vi "database input.vi"(4 "Wheel Name":string="cycle results testdbrunorder.txt", 6 "run number":string="46", 7 "wheelnumber":string, 8 "error in (no error)":errorcluster, 9 "readouts string":string="\r\n1/4/2012 10:09:06 AM\t103752\tWeavCaMB11\tb\tJackson\t0\t3\t50\t1231.000000\tInf\t35.314700\t5.667000\t336.000000\t0.988235\t3599.788248\t31.964787\t6135967.567040\t26573.858939\t1411896.374545\t0.000620\t59.996471\t23532.990455\tNaN\tInf\t0.000000\tNaN\t0.000000\t879579.012026\tNaN\t26573.858939\t0.433083\tNaN\tNaN\tNaN\t7.758172", 10 "runletter":string="testwheellllll", 11 "beamline readbacks":T6={"Injector"=[0.023339, 0.023338, 0.023336000000000003, 0.023338, 0.023336000000000003, 0.023336000000000003, 0.023334], "Analyze"=[0.0058, 0.0058, 0.0058, 0.0058, 0.0058, 0.0058, 0.0058], "Switch"=[0.0, 0.0, 0.0, 0.0, 0.0, 0.0, 0.0], "Terminal"=[0.0010328292846679688, 0.0010328292846679688, 0.0013613700866699219, 0.0007047653198242188, 0.0010328292846679688, 0.0010328292846679688, 0.0010328292846679688], "Cathode"=[10.239062309265137, 10.239218711853027, 10.239218711853027, 10.239218711853027, 10.239218711853027, 10.239218711853027, 10.239218711853027]}) -> (0 "error out":errorcluster={"status"=TRUE, "code"=-2147467259, "source"="NI_Database_API.lvlib:Cmd Execute.vi->NI_Database_API.lvlib:DB Tools Insert Data.vi->database input.vi->2d ams run o17.vi<ERR>ADO Error: 0x80004005\r\nException occured in Microsoft OLE DB Provider for ODBC Drivers: ERROR: invalid input syntax for type double precision: \"True\";\nError while executing the query in NI_Database_API.lvlib:Rec Create - Command.vi->NI_Database_API.lvlib:Cmd Execute.vi->NI_Database_API.lvlib:DB Tools Insert Data.vi->database input.vi->2d ams run o17.vi"}, 1 "db cluster":T5={"startat"="\r\n1/4/2012 10:09:06 AM", "holderid"="103752", "Sample Name"="WeavCaMB11", "type"="b", "User Name"="Jackson", "cycle measured"="0", "position"="3", "estimated ratio"="50", "cycle"="1231.000000", "Transmission"="Inf", "first currents"="35.314700", "runtime"="5.667000", "total rare counts"="336.000000", "livetime"="0.988235", "Rare CPM"="3599.788248", "second current"="31.964787", "17O ratio"="6135967.567040", "17O error"="26573.858939", "Cycle Ratio"="1411896.374545", "cycle error"="0.000620", "interference"="59.996471", "use"="True", "InjSS"="NaN", "He SS"="Inf", "Oaverage"="0.000000", "wheelnumber"="46", "wheel name"="cycle results testdbrunorder.txt", "runnumber"="{0.023339,0.023338,0.023336,0.023338,0.023336,0.023336,0.023334\r\n}", "runletter"="{0.005800,0.005800,0.005800,0.005800,0.005800,0.005800,0.005800\r\n}", "runletter 2"="{0.000000,0.000000,0.000000,0.000000,0.000000,0.000000,0.000000\r\n}"})   [LabVIEW 2016]
doc: "inputs data into cycleresults table in database"
uses:
  controls/db cluster.ctl
  <vilib>/addons/database/Connection.llb/DB Tools Open Connec (String).vi
  <vilib>/addons/database/NI_Database_API.lvlib
panel:
  out "cluster 2":T1
  out "cluster":T2
  out "output cluster 2":T3
  out "output cluster":T4
  in  "db cluster 2":T5={"startat"="\r\n1/4/2012 10:09:06 AM", "holderid"="103752", "Sample Name"="WeavCaMB11", "type"="b", "User Name"="Jackson", "cycle measured"="0", "position"="3", "estimated ratio"="50", "cycle"="1231.000000", "Transmission"="Inf", "first currents"="35.314700", "runtime"="5.667000", "total rare counts"="336.000000", "livetime"="0.988235", "Rare CPM"="3599.788248", "second current"="31.964787", "17O ratio"="6135967.567040", "17O error"="26573.858939", "Cycle Ratio"="1411896.374545", "cycle error"="0.000620", "interference"="59.996471", "use"="True", "InjSS"="NaN", "He SS"="Inf", "Oaverage"="0.000000", "wheelnumber"="46", "wheel name"="cycle results testdbrunorder.txt", "runnumber"="{0.023339,0.023338,0.023336,0.023338,0.023336,0.023336,0.023334\r\n}", "runletter"="{0.005800,0.005800,0.005800,0.005800,0.005800,0.005800,0.005800\r\n}", "runletter 2"="{0.000000,0.000000,0.000000,0.000000,0.000000,0.000000,0.000000\r\n}"}
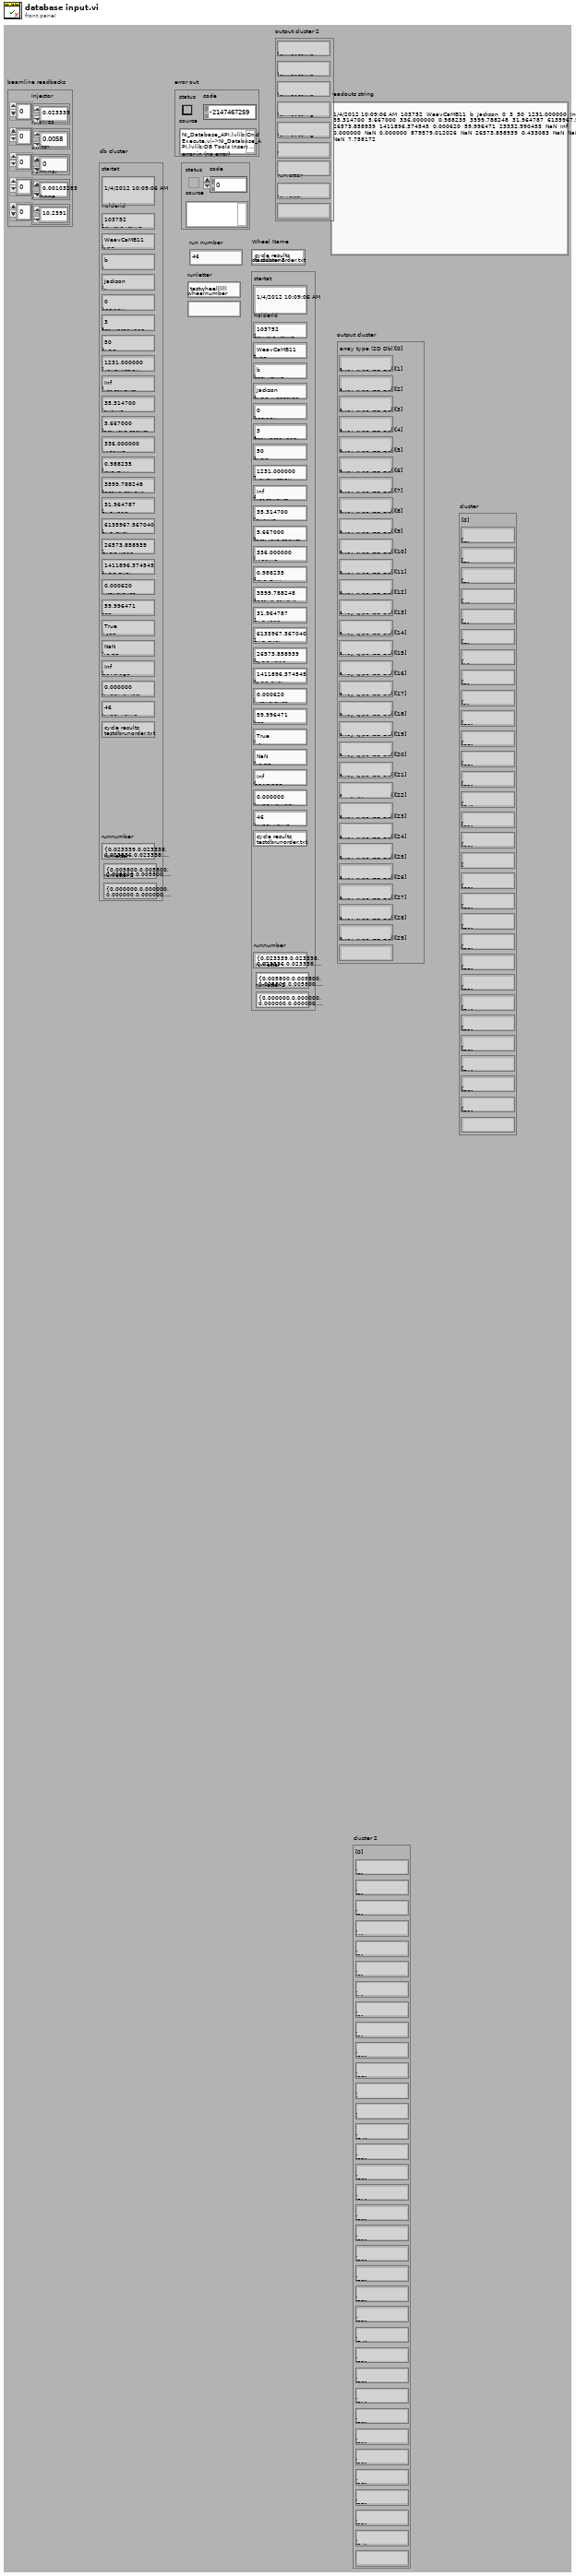
[diagram p1: front panel]
types:
  T1 = cluster{"[0]":string, "[1]":string, "[2]":string, "[3]":string, "[4]":string, "[5]":string, "[6]":string, "[7]":string, "[8]":string, "[9]":string, "[10]":string, "[11]":string, "[12]":string, "[13]":string, "[14]":string, "[15]":string, "[16]":string, "[17]":string, "[18]":string, "[19]":string, "[20]":string, "[21]":string, "[22]":string, "[23]":string, "[24]":string, "[25]":string, "[26]":string, "[27]":string, "[28]":string, "[29]":string, "[30]":string, "[31]":string, "[32]":string, "[33]":string, "[34]":string}
  T2 = cluster{"[0]":string, "[1]":string, "[2]":string, "[3]":string, "[4]":string, "[5]":string, "[6]":string, "[7]":string, "[8]":string, "[9]":string, "[10]":string, "[11]":string, "[12]":string, "[13]":string, "[14]":string, "[15]":string, "[16]":string, "[17]":string, "[18]":string, "[19]":string, "[20]":string, "[21]":string, "[22]":string, "[23]":string, "[24]":string, "[25]":string, "[26]":string, "[27]":string, "[28]":string, "[29]":string}
  T3 = cluster{string, "format string":string, "format string":string, "format string":string, "format string":string, "format string":string, "Wheel Number":string, "runletter":string, "runletter":string}
  T4 = cluster{"array type (2D Dbl)[0]":string, "array type (2D Dbl)[1]":string, "array type (2D Dbl)[2]":string, "array type (2D Dbl)[3]":string, "array type (2D Dbl)[4]":string, "array type (2D Dbl)[5]":string, "array type (2D Dbl)[6]":string, "array type (2D Dbl)[7]":string, "array type (2D Dbl)[8]":string, "array type (2D Dbl)[9]":string, "array type (2D Dbl)[10]":string, "array type (2D Dbl)[11]":string, "array type (2D Dbl)[12]":string, "array type (2D Dbl)[13]":string, "array type (2D Dbl)[14]":string, "array type (2D Dbl)[15]":string, "array type (2D Dbl)[16]":string, "array type (2D Dbl)[17]":string, "array type (2D Dbl)[18]":string, "array type (2D Dbl)[19]":string, "array type (2D Dbl)[20]":string, "array type (2D Dbl)[21]":string, "array type (2D Dbl)[22]":string, "array type (2D Dbl)[23]":string, "array type (2D Dbl)[24]":string, "array type (2D Dbl)[25]":string, "array type (2D Dbl)[26]":string, "array type (2D Dbl)[27]":string, "array type (2D Dbl)[28]":string, "array type (2D Dbl)[29]":string}
  T5 = typedef "db cluster.ctl" = cluster{"startat":string, "holderid":string, "Sample Name":string, "type":string, "User Name":string, "cycle measured":string, "position":string, "estimated ratio":string, "cycle":string, "Transmission":string, "first currents":string, "runtime":string, "total rare counts":string, "livetime":string, "Rare CPM":string, "second current":string, "17O ratio":string, "17O error":string, "Cycle Ratio":string, "cycle error":string, "interference":string, "use":string, "InjSS":string, "He SS":string, "Oaverage":string, "wheelnumber":string, "wheel name":string, "runnumber":string, "runletter":string, "runletter 2":string}
  T6 = cluster{"Injector":dbl[], "Analyze":dbl[], "Switch":dbl[], "Terminal":dbl[], "Cathode":dbl[]}
  T7 = cluster{string, "format string":string, "format string":string, "format string":string, "format string":string, "format string":string, "wheelnumber":string, "runletter":string, "run number":string}
  T8 = typedef "NI_Database_API.lvlib/Conn ObjectReference.ctl" = refnum<k1>
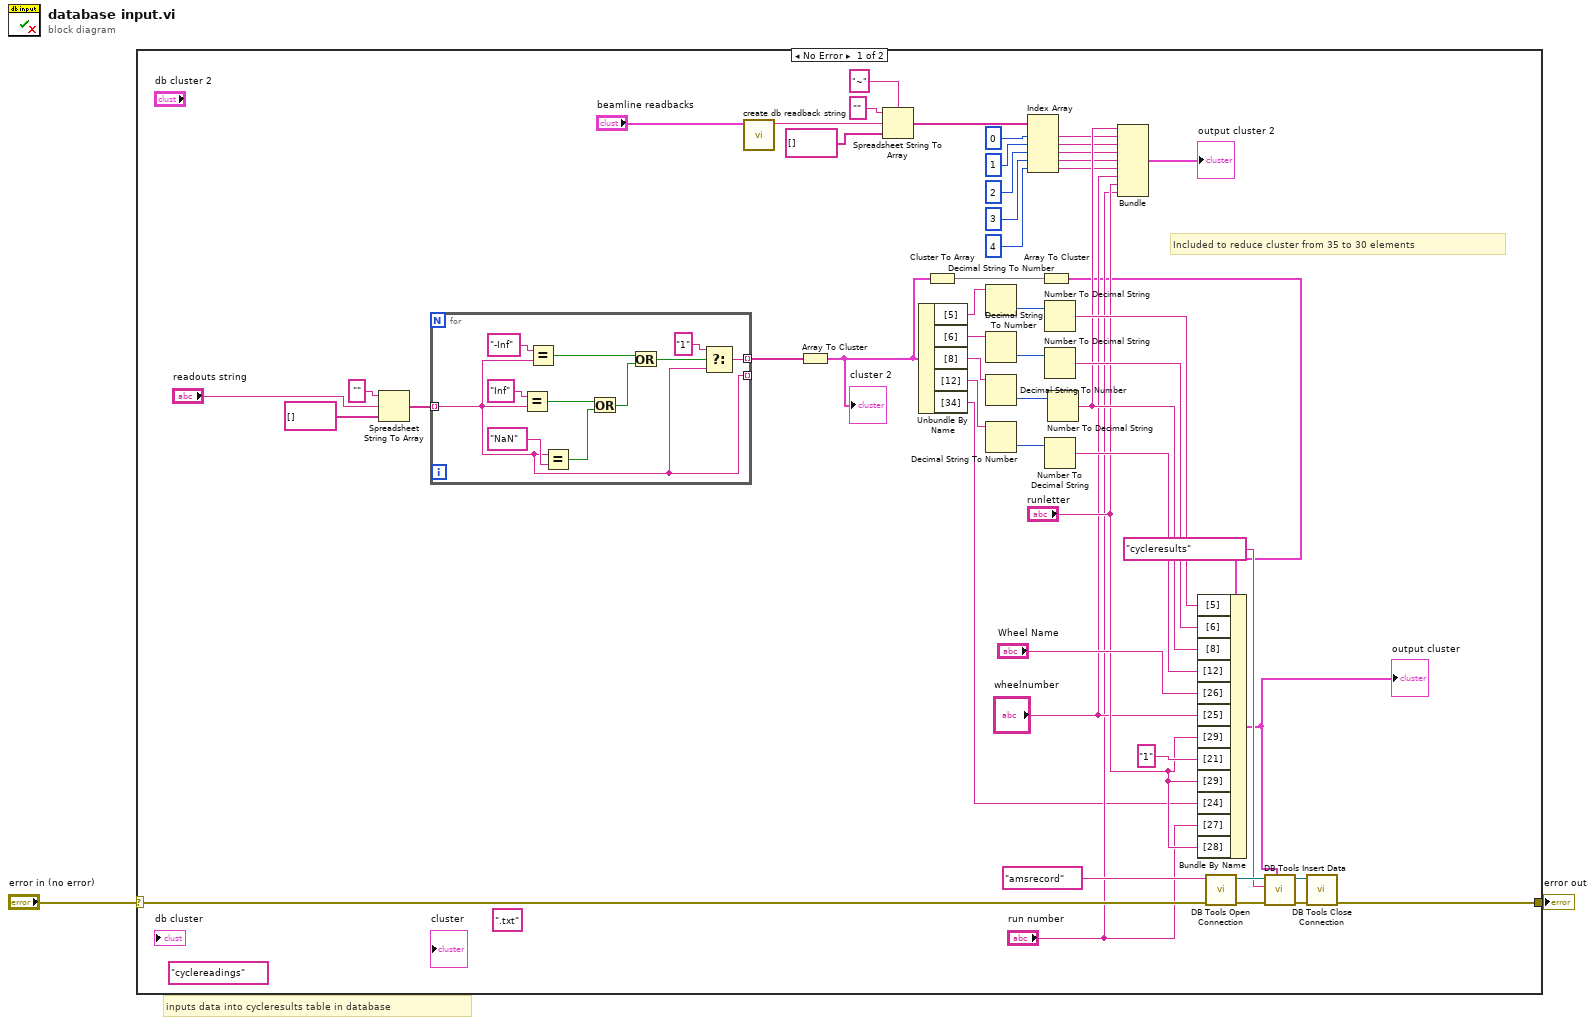
[diagram p0: block diagram]
diagram:
  # "inputs data into cycleresults table in database"
  n1 = case shown="No Error" "error in (no error)" {
    selector: "error in (no error)" -> [w43 w66]
    tunnel: [w29 w66] -> w2
    frame No Error {
      (unwired) "cyclereadings" ("table")
      (unwired) ".txt" ("regular expression")
      # "Included to reduce cluster from 35 to 30 elements"
      n2 = Spreadsheet String To Array(format string="", spreadsheet string="readouts string", array type (2D Dbl)=string[] []) -> (array=w12:string[])  [unwired: 1 in]
      n3 = for {
        tunnel: [w58] -> _ mode=indexing
        tunnel: [w60] -> w10 mode=indexing
        tunnel: w12 -> [w58] mode=indexing
        n4 = Equal?(x="Inf" ("y"), y=w58) -> (x = y?=w63:bool)
        n5 = Equal?(x="-Inf" ("y"), y=w58) -> (x = y?=w57:bool)
        n6 = Equal?(x=w58, y="NaN") -> (x = y?=w62:bool)
        n7 = Or(x=w63, y=w62) -> (x .or. y?=w56:bool)
        n8 = Or(x=w57, y=w56) -> (x .or. y?=w55:bool)
        n9 = Select(t="1", s=w55, f=w58) -> (s? t:f=w60:string)
      }
      n10 = call "create db readback string.vi"("beamline readbacks"="beamline readbacks") -> ("arry of readback strings"=w45:string)  [unwired: 9 in, 1 out]
      n11 = Array To Cluster(array=w10) -> (cluster=w8:T1)
      "cluster 2" <- w8
      n12 = Spreadsheet String To Array(delimiter (Tab)="~", format string="", spreadsheet string=w45, array type (2D Dbl)=string[] []) -> (array=w27:string[])
      n13 = Unbundle By Name(w8) -> ("[5]"=w41:string, "[6]"=w40:string, "[8]"=w36:string, "[12]"=w35:string, "[34]"=w9:string)
      n14 = Cluster To Array(cluster=w8) -> (array=w7:string[])
      n15 = Decimal String To Number(string=w41) -> (number=w31:i32)  [unwired: 2 in, 1 out]
      n16 = Decimal String To Number(string=w40) -> (number=w32:i32)  [unwired: 2 in, 1 out]
      n17 = Decimal String To Number(string=w36) -> (number=w37:i32)  [unwired: 2 in, 1 out]
      n18 = Decimal String To Number(string=w35) -> (number=w34:i32)  [unwired: 2 in, 1 out]
      n19 = Index Array(array=w27, index #1=0 ("index"), index #2=1 ("index"), index #3=2 ("index"), index #4=3 ("index"), index #5=4 ("index")) -> (element #1=w25:string, element #2=w23:string, element #3=w21:string, element #4=w19:string, element #5=w17:string)
      n20 = Array To Cluster(array=w7) -> (cluster=w6:T2)
      n21 = Number To Decimal String(number=w31) -> (decimal integer string=w39:string)  [unwired: 1 in]
      n22 = Number To Decimal String(number=w32) -> (decimal integer string=w38:string)  [unwired: 1 in]
      n23 = Number To Decimal String(number=w34) -> (decimal integer string=w33:string)  [unwired: 1 in]
      n24 = Number To Decimal String(number=w37) -> (decimal integer string=w28:string)  [unwired: 1 in]
      n25 = Bundle(w28, "format string"=w25, "format string"=w23, "format string"=w21, "format string"=w19, "format string"=w17, "wheelnumber"="wheelnumber", "runletter"="runletter", "run number"="run number") -> (→"output cluster 2":T7)  [unwired: 1 in]
      n26 = Bundle By Name(cluster=w6, "[5]"=w39, "[6]"=w38, "[8]"=w28, "[12]"=w33, "[26]"="Wheel Name", "[25]"="wheelnumber", "[29]"="runletter", "[21]"="1" ("format string"), "[29]"="runletter", "[24]"=w9, "[27]"="run number", "[28]"="runletter") -> (w5:T2)
      "output cluster" <- w5
      n27 = call-poly <vilib>:"DB Tools Open Connection.vi"("error in (no error)"=w43, "connection information"="amsrecord") -> ("error out"=w53:errorcluster, "connection reference"=w54:T8)  [unwired: 6 in]
      n28 = call <vilib>:"DB Tools Insert Data.vi"("data"=w5, "error in (no error)"=w53, "table"="cycleresults" ("String"), "connection reference"=w54) -> ("error out"=w3:errorcluster, "connection reference out"=w4:T8)  [unwired: 6 in]
      n29 = call <vilib>:"DB Tools Close Connection.vi"("error in (no error)"=w3, "connection reference"=w4) -> ("error out"=w29:errorcluster)  [unwired: 5 in]
    }
    frame Error {
    }
  }
  "error out" <- w2
